vi "ABCD free space dist.vi"(1 "Dist":dbl format="%.2f") -> (0 "ABCD":cluster{"A":dbl, "B":dbl, "C":dbl, "D":dbl} {"D" format="%.2f"; "C" format="%.2f"; "B" format="%.2f"; "A" format="%.2f"})   [LabVIEW 2017]
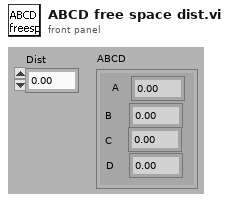
[diagram p1: front panel]
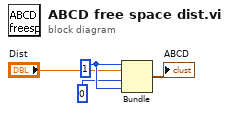
[diagram p0: block diagram]
diagram:
  w3 = 1
  n1 = Bundle(w3, "Dist"="Dist", "Index (row)"=0, w3) -> (→"ABCD":cluster{i32, "Dist":dbl, "Index (row)":i32, i32})  [unwired: 1 in]
